vi "ModeFieldOriented.vi"() -> (0 "Orientation Mode":enum16{"Robot-Oriented", "Field-Oriented"}(ring))   [LabVIEW 2019]
doc: "This VI manages whether the swerve drive is in robot-oriented or field-oriented mode, based on driver inputs, emergency overrides, and safety interlocks."
uses:
  sensors.vi
  dsdata.vi
  outputs.vi
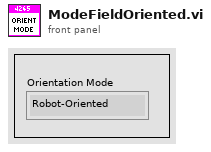
[diagram p1: front panel]
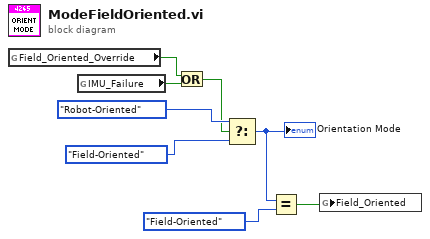
[diagram p0: block diagram]
diagram:
  n1 = global read "dsdata.vi" "Field_Oriented_Override"() -> (w3:bool)
  n2 = global read "sensors.vi" "IMU_Failure"() -> (w4:bool)
  n3 = Or(x=w3, y=w4) -> (x .or. y?=w2:bool)
  n4 = Select(t=enum16{"Robot-Oriented", "Field-Oriented"}."Robot-Oriented", s=w2, f=enum16{"Robot-Oriented", "Field-Oriented"}."Field-Oriented") -> (s? t:f=w8:enum16{"Robot-Oriented", "Field-Oriented"})
  "Orientation Mode" <- w8
  n5 = Equal?(x=w8, y=enum16{"Robot-Oriented", "Field-Oriented"}."Field-Oriented") -> (x = y?=w7:bool)
  n6 = global write "outputs.vi" "Field_Oriented"(w7) -> ()
